vi "Connect.vi"(8 "error in (no error)":errorcluster, 10 "Connection list in":string, 11 "Abstract Switch Consumer in":refnum<class "Abstract Switch Consumer.lvclass">) -> (0 "error out":errorcluster, 3 "Abstract Switch Consumer out":refnum<class "Abstract Switch Consumer.lvclass">)   [LabVIEW 2027, in "Messaging.lvlib" / "Abstract Switch Consumer.lvclass"]
uses:
  Abstract Switch Consumer.lvclass
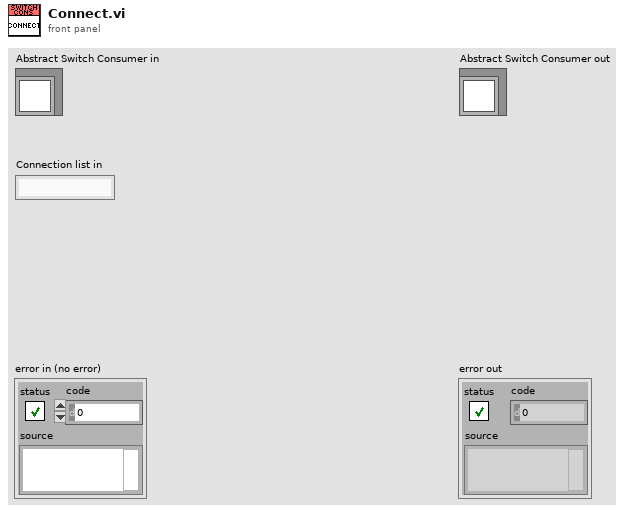
[diagram p1: front panel]
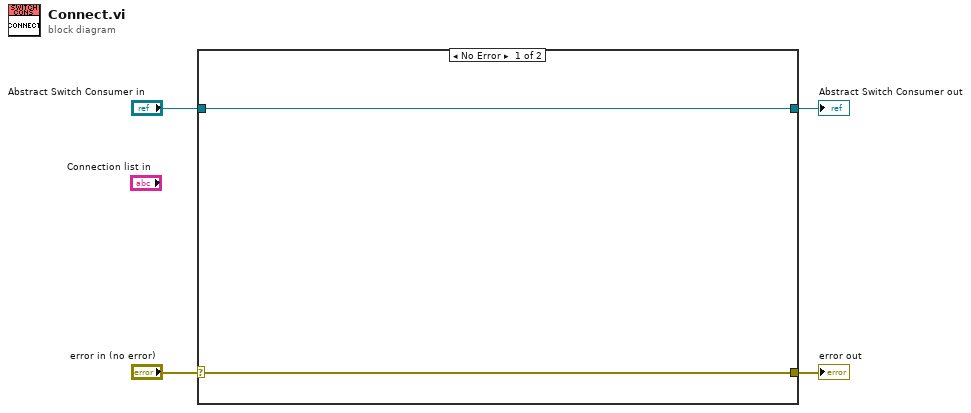
[diagram p0: block diagram]
diagram:
  n1 = case shown="No Error" "error in (no error)" {
    selector: "error in (no error)" -> [w5 w8]
    tunnel: [w5 w8] -> w3
    tunnel: [w6 w7] -> w1
    tunnel: "Abstract Switch Consumer in" -> [w6 w7]
    frame No Error {
    }
    frame Error {
    }
  }
  "error out" <- w3
  "Abstract Switch Consumer out" <- w1
